vi "ExternalProcessTemplate.vi"(10 "InitString":string, 11 "EVE reference in":refnum<data-value>) -> ()   [LabVIEW 2013]
uses:
  001 - MAIN/Class/EVE/EVE.lvclass
  090 - ERRORS/Ctrls/enumLogAndView.ctl
  030 - EVENTS/EnumFgvEventCommand.ctl
  030 - EVENTS/03 - ToMessageHandlerProcess/ToMessageHandlerEvent.ctl
  030 - EVENTS/03 - ToMessageHandlerProcess/enumMessageCriticity.ctl
panel:
  # "Template de process externe..."
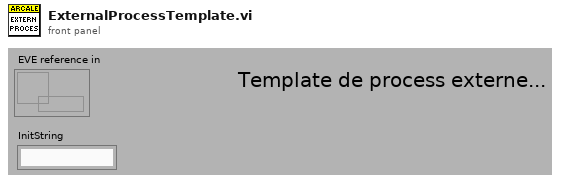
[diagram p1: front panel]
types:
  T1 = typedef "enumLogAndView.ctl" = enum16{"Log only", "Log and view"}
  T2 = typedef "EnumFgvEventCommand.ctl" = enum16{"Setup", "Cleanup", "Get"}
  T3 = typedef "enumMessageCriticity.ctl" = enum16{"No error", "Info", "Warning", "Error", "Fatal error"}
  T4 = typedef "ToMessageHandlerEvent.ctl" = cluster{"date / time":timestamp, "Criticity":T3, "Emitter":string, "Message":string}
  T5 = enum32{"Invalid", "Standard", "Closed", "Hidden", "Minimized", "Maximized"}
  T6 = typedef "EnumToAllProcessesCommand.ctl" = enum16{"Stop all processes", "Autotest"}
  T7 = typedef "ToProcess_EnumCommand.ctl" = enum16{"Show front panel", "Hide front panel"}
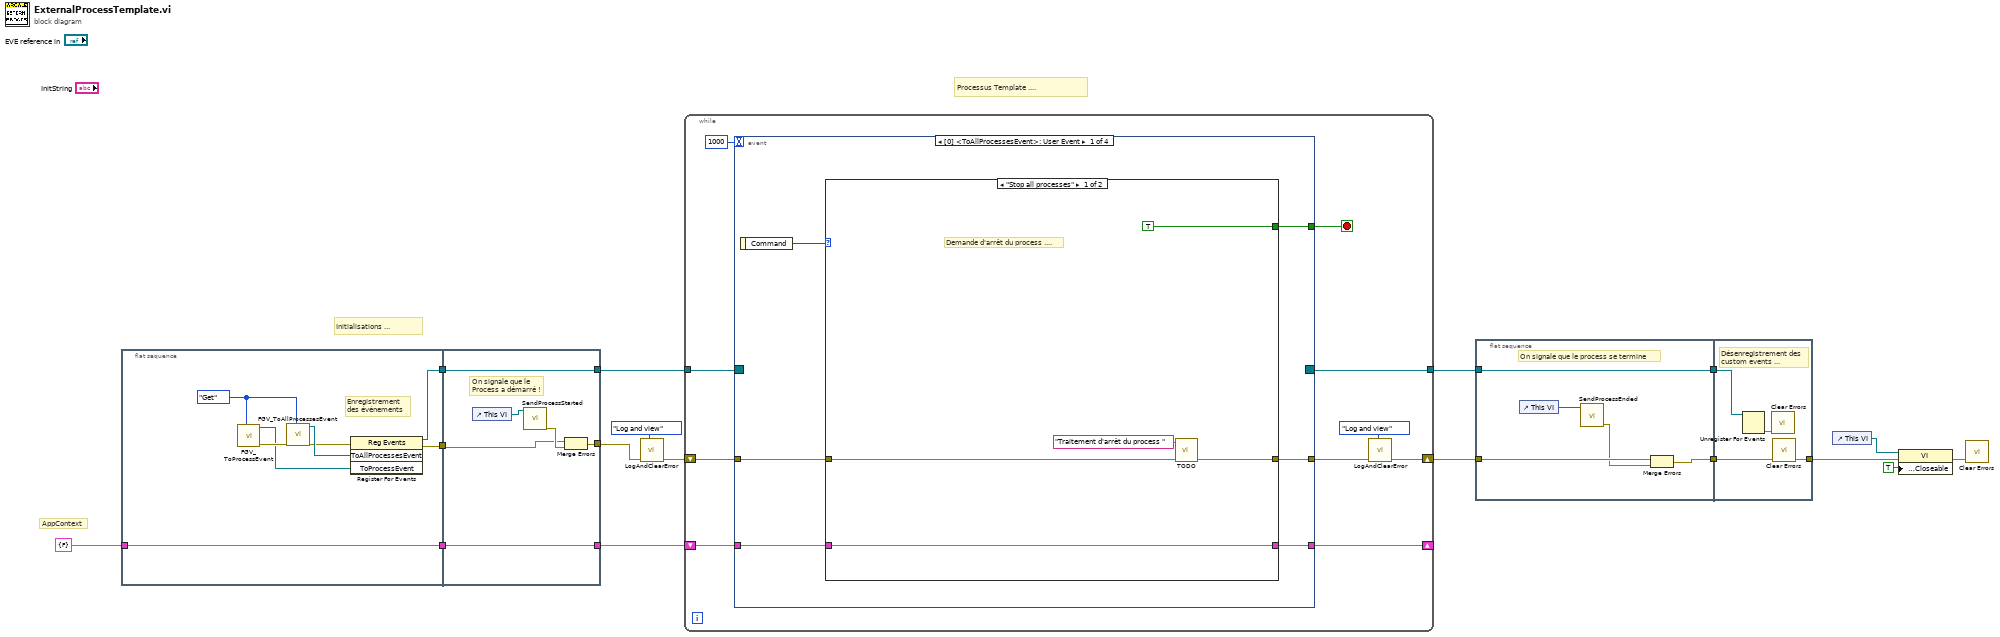
[diagram p0: block diagram]
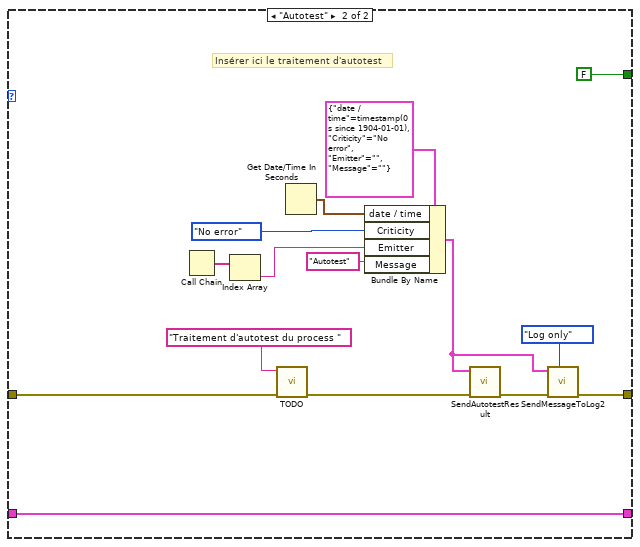
[diagram p2: hidden frame]
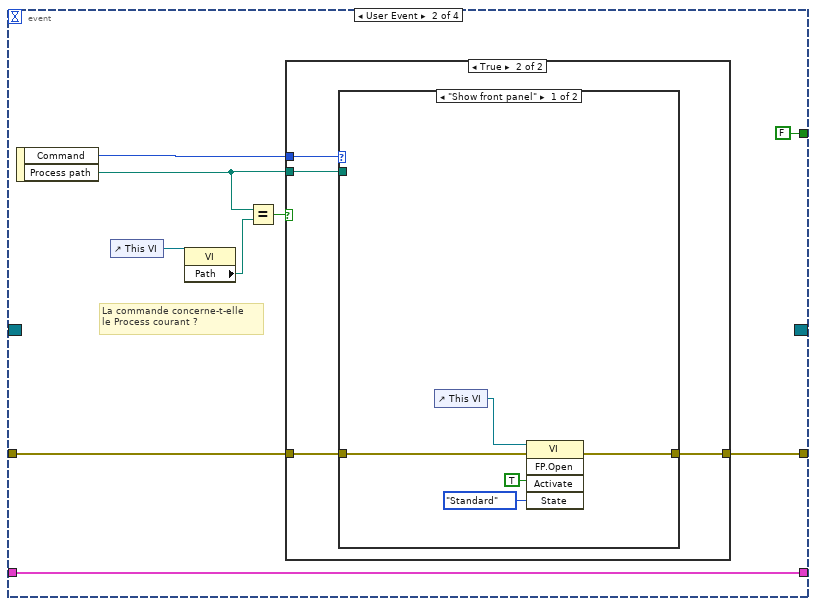
[diagram p3: hidden frame]
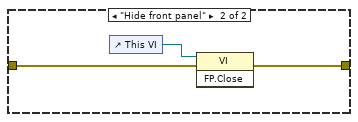
[diagram p5: hidden frame]
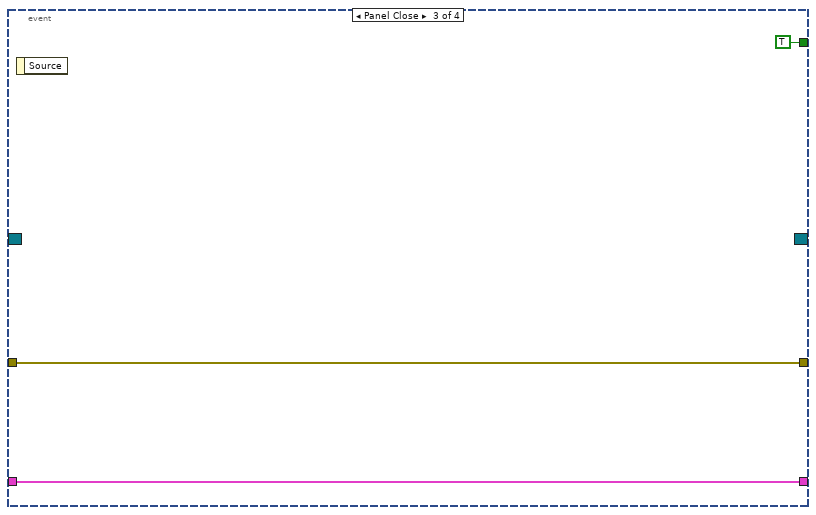
[diagram p6: hidden frame]
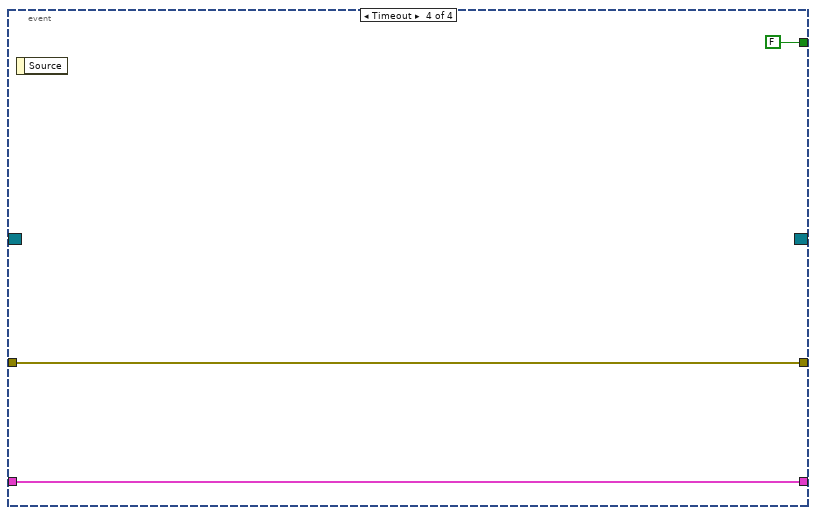
[diagram p7: hidden frame]
diagram:
  # "AppContext"
  # "Initialisations ..."
  # "Processus Template ...."
  n1 = flat-sequence {
    tunnel: cluster{"Boolean":bool} {"Boolean"=FALSE} ("AppContext") -> [w25]
    tunnel: [w25] -> w13
    tunnel: [w22] -> w8
    tunnel: [w21] -> w7
    tunnel: [w31] -> w9
    tunnel: [w28] -> w17
    tunnel: w13 -> [w30]
    tunnel: [w30] -> w12
    tunnel: w8 -> [w27]
    tunnel: w7 -> [w28]
    frame #0 {
      w20 = EnumFgvEventCommand."Get" ("Command")
      # "Enregistrement \ndes événements"
      n2 = call "FGV_ToProcessEvent.vi"("Command"=w20) -> ("error out"=w19:errorcluster, "ToProcessEvent"=w18:refnum<user-event>)  [unwired: 9 in]
      n3 = call "FGV_ToAllProcessesEvent.vi"("Command"=w20, "error in (no error)"=w19) -> ("error out"=w23:errorcluster, "ToAllProcessesEvent"=w24:refnum<user-event>)  [unwired: 8 in]
      n4 = register-events(error in=w23, w24, w18) -> (reference out=w21:refnum<event-registration>, error out=w22:errorcluster)  [unwired: 1 in]
    }
    frame #1 {
      # "On signale que le\nProcess a démarré !"
      n5 = control-ref of="This VI"() -> (w26:refnum<vi>)
      n6 = call "SendProcessStarted.vi"("Process Refnum"=w26) -> ("error out"=w29:errorcluster)  [unwired: 10 in]
      n7 = Merge Errors(w27, w29) -> (w31:errorcluster)
    }
  }
  n8 = call "LogAndClearError.vi"("Log and view ?"=enumLogAndView."Log and view", "error in (no error)"=w9) -> ("error out"=w10:errorcluster)  [unwired: 9 in]
  n9 = while {
    shift-right: [w35] -> w15
    shift-left: w10 -> [w32]
    tunnel: w17 -> [w41]
    tunnel: [w40] -> w16
    shift-right: [w37] -> _
    shift-left: w12 -> [w38]
    stop <- w39 stop-if-true
    n10 = event shown="[0] <ToAllProcessesEvent>: User Event" {
      selector: w41 -> [_ _ _ _]
      dyn-events: [_ _ _ _] -> w40
      timeout: 1000 -> [_ _ _ _]
      tunnel: w32 -> [w45 w75 w91 w95]
      tunnel: [w44 w71 w91 w95] -> w36
      tunnel: [w46 FALSE TRUE FALSE] -> w39
      tunnel: w38 -> [w43 w70 w90 w94]
      tunnel: [w42 w70 w90 w94] -> w37
      event User Event {
        n11 = event-data() -> ("Command"=w47:T6)  [unwired: 1 in]
        n12 = case shown="\"Stop all processes\"" w47 {
          tunnel: [TRUE FALSE] -> w46
          tunnel: w45 -> [w48 w64]
          tunnel: [w50 w55] -> w44
          tunnel: w43 -> [w51 w67]
          tunnel: [w51 w67] -> w42
          frame "Stop all processes" {
            # "Demande d'arrêt du process ...."
            n13 = call "TODO.vi"("error in (no error)"=w48, "Message"="Traitement d'arrêt du process ") -> ("error out"=w50:errorcluster)  [unwired: 9 in]
          }
          frame "Autotest" {
            # "Insérer ici le traitement d'autotest"
            n14 = Call Chain() -> (call chain=w59:string[])
            n15 = Index Array(array=w59) -> (element=w58:string)  [unwired: 1 in]
            n16 = call "TODO.vi"("error in (no error)"=w64, "Message"="Traitement d'autotest du process ") -> ("error out"=w63:errorcluster)  [unwired: 9 in]
            n17 = Get Date/Time In Seconds() -> (seconds since 1Jan1904=w61:timestamp)
            n18 = Bundle By Name(cluster=T4 {"date / time"=timestamp(0 s since 1904-01-01), "Criticity"=enum."No error", "Emitter"="", "Message"=""} ("Message"), "date / time"=w61, "Criticity"=enumMessageCriticity."No error", "Emitter"=w58, "Message"="Autotest") -> (w54:T4)
            n19 = call "SendAutotestResult.vi"("error in (no error)"=w63, "Message"=w54) -> ("error out"=w56:errorcluster)  [unwired: 9 in]
            n20 = call "SendMessageToLog2.vi"("Log and view ?"=enumLogAndView."Log only", "error in (no error)"=w56, "Message"=w54) -> ("error out"=w55:errorcluster)  [unwired: 8 in]
          }
        }
      }
      event User Event {
        # "La commande concerne-t-elle\nle Process courant ?"
        n21 = event-data() -> ("Command"=w76:T7, "Process path"=w73:path)  [unwired: 1 in]
        n22 = control-ref of="This VI"() -> (w74:refnum<vi>)
        n23 = property class="VI"(reference=w74) -> ("Path"=w72:path)  [unwired: 1 in, 2 out]
        n24 = Equal?(x=w73, y=w72) -> (x = y?=w69:bool)
        n25 = case shown="True" w69 {
          tunnel: w76 -> [_ w81]
          tunnel: w75 -> [w77 w80]
          tunnel: w73 -> [_ w79]
          tunnel: [w77 w78] -> w71
          frame False {
            # "La commande n'est pas pour ce process !"
          }
          frame True {
            n26 = case shown="\"Show front panel\"" w81 {
              tunnel: w80 -> [w85 w88]
              tunnel: w79 -> [_ _]
              tunnel: [w84 w87] -> w78
              frame "Show front panel" {
                n27 = control-ref of="This VI"() -> (w86:refnum<vi>)
                n28 = invoke class="VI" method="FP.Open"(reference=w86, error in=w85, "Activate"=TRUE ("Activate?"), "State"=T5."Standard") -> (error out=w84:errorcluster)  [unwired: 1 in, 4 out]
              }
              frame "Hide front panel" {
                n29 = control-ref of="This VI"() -> (w89:refnum<vi>)
                n30 = invoke class="VI" method="FP.Close"(reference=w89, error in=w88) -> (error out=w87:errorcluster)  [unwired: 1 in, 2 out]
              }
            }
          }
        }
      }
      event Panel Close {
        n31 = event-data() -> ()  [unwired: 1 in, 1 out]
      }
      event Timeout {
        n32 = event-data() -> ()  [unwired: 1 in, 1 out]
      }
    }
    n33 = call "LogAndClearError.vi"("Log and view ?"=enumLogAndView."Log and view", "error in (no error)"=w36) -> ("error out"=w35:errorcluster)  [unwired: 9 in]
  }
  n34 = flat-sequence {
    tunnel: w15 -> [w99]
    tunnel: w16 -> [w100]
    tunnel: [w100] -> w2
    tunnel: [w97] -> w1
    tunnel: [w101] -> w6
    tunnel: w2 -> [w104]
    tunnel: w1 -> [w102]
    frame #0 {
      # "On signale que le process se termine"
      n35 = control-ref of="This VI"() -> (w96:refnum<vi>)
      n36 = call "SendProcessEnded.vi"("Process Refnum"=w96) -> ("error out"=w98:errorcluster)  [unwired: 10 in]
      n37 = Merge Errors(w99, w98) -> (w97:errorcluster)
    }
    frame #1 {
      # "Désenregistrement des\ncustom events ..."
      n38 = Unregister For Events(event registration refnum=w104) -> (error out=w103:errorcluster)  [unwired: 1 in]
      n39 = call <vilib>:"Clear Errors.vi"("error in (no error)"=w103) -> ()  [unwired: 6 in, 1 out]
      n40 = call <vilib>:"Clear Errors.vi"("error in (no error)"=w102) -> ("error out"=w101:errorcluster)  [unwired: 6 in]
    }
  }
  n41 = control-ref of="This VI"() -> (w5:refnum<vi>)
  n42 = property class="VI"(reference=w5, error in=w6, "Front Panel.Closeable"=TRUE ("Front Panel Window:Closeable")) -> (error out=w3:errorcluster)  [unwired: 1 out]
  n43 = call <vilib>:"Clear Errors.vi"("error in (no error)"=w3) -> ()  [unwired: 6 in, 1 out]
